vi "Get Storage Size.vi"(11 "PN532 COM Port":refnum<visa-resource-name>) -> (0 "error out":errorcluster, 2 "Storage Size":i32, 3 "PN532 COM Port out":refnum<visa-resource-name>)   [LabVIEW 2012, in "NFC Driver.lvlib"]
uses:
  NFC Driver.lvlib
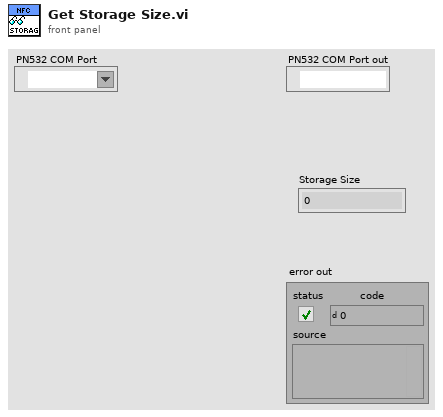
[diagram p1: front panel]
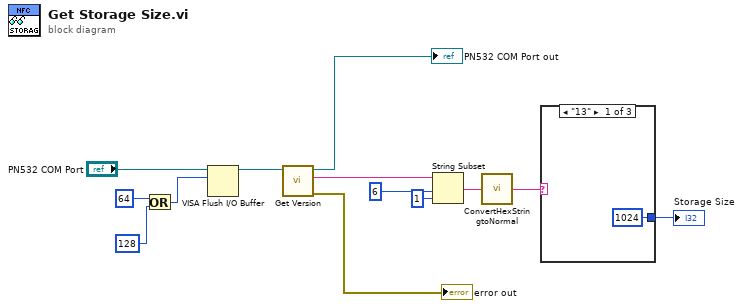
[diagram p0: block diagram]
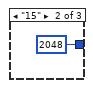
[diagram p2: hidden frame]
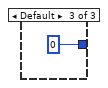
[diagram p3: hidden frame]
diagram:
  n1 = Or(x=64, y=128) -> (x .or. y?=w4:i32)
  n2 = VISA Flush I/O Buffer(VISA resource name="PN532 COM Port", mask (16)=w4) -> (VISA resource name out=w2:refnum<visa-resource-name>)  [unwired: 1 in, 1 out]
  n3 = call "Get Version.vi"("PN532 COM Port"=w2) -> ("error out"=→"error out":errorcluster, "Version Data"=w3:string, "PN532 COM Port"=→"PN532 COM Port out":refnum<visa-resource-name>)  [unwired: 8 in]
  n4 = String Subset(string=w3, offset (0)=6, length (rest)=1 ("length (rest)")) -> (substring=w10:string)
  n5 = call "ConvertHexStringtoNormal.vi"("Hex String"=w10) -> ("Normal String"=w9:string)
  n6 = case shown="\"13\"" w9 {
    tunnel: [1024 2048 ("Storage Size") 0 ("Storage Size")] -> w8
    frame "13" {
    }
    frame "15" {
    }
    frame Default {
    }
  }
  "Storage Size" <- w8
